vi "RTCurveStart.vi"(11 "Queue in":refnum<queue>) -> ()   [LabVIEW 2020]
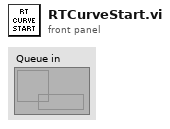
[diagram p1: front panel]
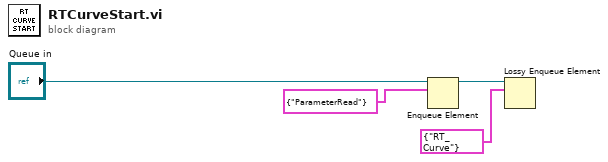
[diagram p0: block diagram]
diagram:
  n1 = Enqueue Element(queue="Queue in", element=cluster{"Command":string} {"Command"="ParameterRead"}) -> (queue out=w3:refnum<queue>)  [unwired: 2 in, 2 out]
  n2 = Lossy Enqueue Element(queue=w3, element=cluster{"Command":string} {"Command"="RT_Curve"}) -> ()  [unwired: 1 in, 4 out]
